vi "FRCts20_WebMethods_Convert_Requests.vi"(8 "error in (no error)":errorcluster, 11 "Request":T3) -> (0 "error out":errorcluster, 3 "output cluster":T1)   [LabVIEW 2014, in "FRCts20_WebMethods.lvlib"]
uses:
  FRCts20_WebMethods.lvlib
  Backend/source/VI Source/FRCts20_Backend_API/FRCts20_Backend_API_Status.ctl
  Backend/source/VI Source/FRCts20_Backend_API/FRCts20_Backend_API_RequestRoot.ctl
  Web Method Public Interface/FRCts20_WebMethods_ctl_request.ctl
  Backend/source/VI Source/FRCts20_Backend_API/FRCts20_Backend_API.lvlib
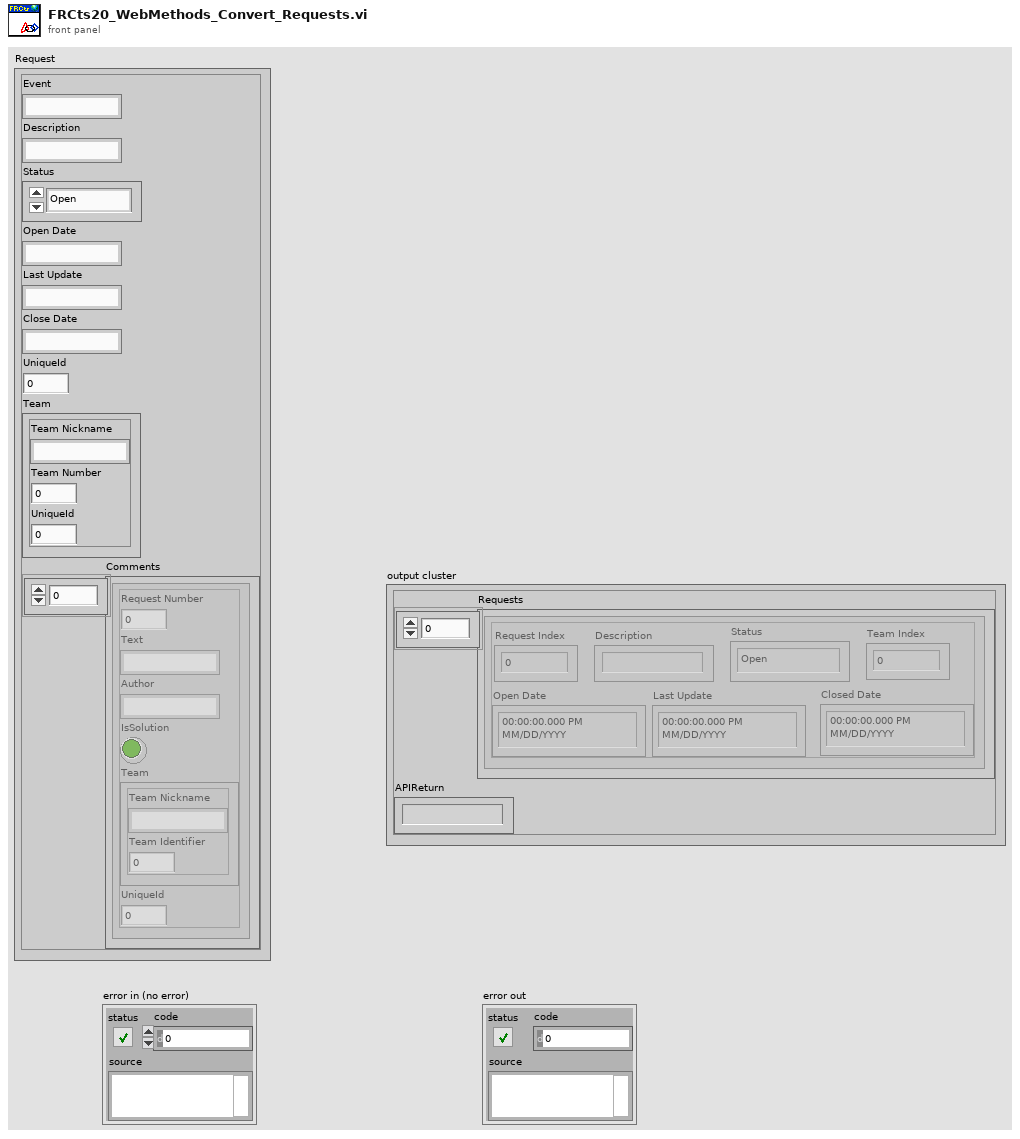
[diagram p1: front panel]
types:
  T1 = typedef "FRCts20_Backend_API.lvlib/FRCts20_Backend_API_RequestRoot.ctl" = cluster{"Requests":cluster{"Request Index":u32, "Description":string, "Status":T2, "Open Date":timestamp, "Last Update":timestamp, "Closed Date":timestamp, "Team Index":u32}[], "APIReturn":string}
  T2 = typedef "FRCts20_Backend_API.lvlib/FRCts20_Backend_API_Status.ctl" = enum16{"Open", "In Work", "Closed"}
  T3 = typedef "FRCts20_WebMethods.lvlib/FRCts20_WebMethods_ctl_request.ctl" = cluster{"Event":string, "Description":string, "Status":T4, "Open Date":string, "Last Update":string, "Close Date":string, "UniqueId":i32, "Team":cluster{"Team Nickname":string, "Team Number ":i32, "UniqueId":i32}, "Comments":cluster{"Request Number":dbl, "Text":string, "Author":string, "IsSolution":bool, "Team":cluster{"Team Nickname":string, "Team Identifier ":dbl}, "UniqueId":i32}[]}
  T4 = typedef "FRCts20_Backend_Engine.lvlib/FRCts20_Backend_API.lvlib/FRCts20_Backend_API_Status.ctl" = enum16{"Open", "In Work", "Closed"}
  T5 = cluster{"Request Index":u32, "Description":string, "Status":T2, "Open Date":timestamp, "Last Update":timestamp, "Closed Date":timestamp, "Team Index":u32}
  T6 = cluster{"Request Index":u32, "Description":string, "Status":T2, "Open Date":timestamp, "Last Update":timestamp, "Closed Date":timestamp, "Team Index":u32}[]
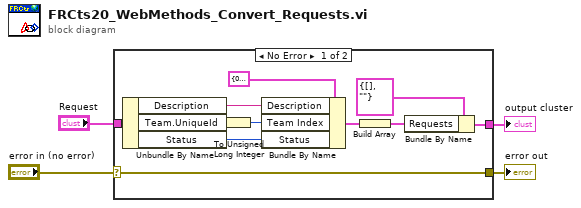
[diagram p0: block diagram]
diagram:
  n1 = case shown="No Error" "error in (no error)" {
    selector: "error in (no error)" -> [w15 w16]
    tunnel: [w5 _] -> w1
    tunnel: "Request" -> [w14 _]
    tunnel: [w15 w16] -> w4
    frame No Error {
      n2 = Unbundle By Name(w14) -> ("Description"=w13:string, "Team.UniqueId"=w11:i32, "Status"=w12:T4)
      n3 = To Unsigned Long Integer(number=w11) -> (unsigned 32bit integer=w10:u32)
      n4 = Bundle By Name(cluster=T5 {"Request Index"=0, "Description"="", "Status"=enum."Open", "Open Date"=timestamp(0 s since 1904-01-01), "Last Update"=timestamp(0 s since 1904-01-01), "Closed Date"=timestamp(0 s since 1904-01-01), "Team Index"=0} ("Request 3"), "Description"=w13, "Team Index"=w10, "Status"=w12) -> (w7:T5)
      n5 = Build Array(w7) -> (w6:T6)
      n6 = Bundle By Name(cluster=T1 {"Requests"=[], "APIReturn"=""} ("Request In"), "Requests"=w6) -> (w5:T1)
    }
    frame Error {
    }
  }
  "error out" <- w4
  "output cluster" <- w1
